vi "GetOutputShapeDimCount.vi"(8 "error in (no error)":errorcluster, 10 "outputIndex":i32, 11 "session id in":i32) -> (0 "error out":errorcluster, 2 "OutputShapeDimCount":i32, 3 "session id out":i32)   [LabVIEW 2017, in "libonnx_wrapper.lvlib"]
doc: "/**\n * @brief Получить количество размерностей выходного тензора\n * \n * Возвращает ранг тензора (число измерений). Например:\n * - Вектор [10] имеет 1 размерность\n * - Матрица [1, 10] имеет 2 размерности\n * - Изображение [1, 3, 224, 224] имеет 4 размерности\n * \n * @param sessionId [IN] ID сессии\n * @param outputIndex [IN] Индекс входа (0-based)\n * \n * @return int32: Количество размерностей (1, 2, 3, 4, ...)\n * @return int32: 0 если сессия не найдена или индекс неверен\n */\nint GetOutputShapeDimCount(int sessionId, int outputIndex);"
uses:
  libonnx_wrapper.lvlib
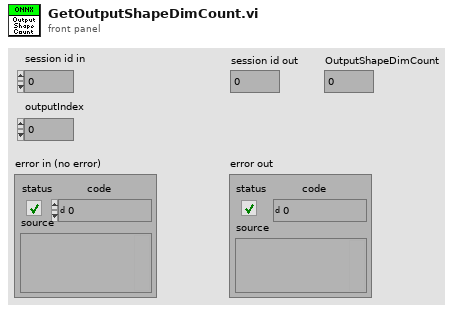
[diagram p1: front panel]
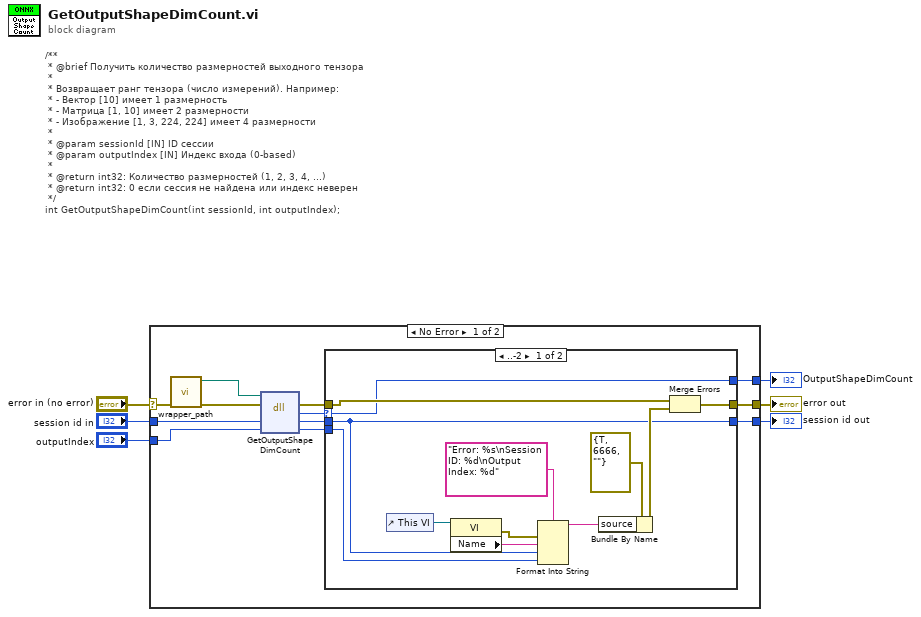
[diagram p0: block diagram]
diagram:
  # "/**\n * @brief Получить количество размерностей выходного тензора\n * \n * Возвращает ранг тензора (число измерений). Например:\n * - Вектор [10] имеет 1 размерность\n * - Матрица [1, 10] имеет 2 размерности\n * - Изображение [1, 3, 224, 224] имеет 4 размерности\n * \n * @param sessionId [IN] ID сессии\n * @param outputIndex [IN] Индекс входа (0-based)\n * \n * @return int32: Количество размерностей (1, 2, 3, 4, ...)\n * @return int32: 0 если сессия не найдена или индекс неверен\n */\nint GetOutputShapeDimCount(int sessionId, int outputIndex);"
  n1 = case shown="No Error" "error in (no error)" {
    selector: "error in (no error)" -> [w7 w35]
    tunnel: "outputIndex" -> [w18 _]
    tunnel: "session id in" -> [w16 w34]
    tunnel: [w13 w35] -> w4
    tunnel: [w11 _] -> w3
    tunnel: [w10 w34] -> w2
    frame No Error {
      n2 = call "wrapper_path.vi"("error in (no error)"=w7) -> ("error out"=w15:errorcluster, "wrapper path"=w17:path)  [unwired: 9 in]
      n3 = dll-call lib="home/ivan/LabVIEWData/ONNX/Test/libonnx_wrapper/unix64/libonnx_wrapper.so" fn="GetOutputShapeDimCount"(path in=w17, error in=w15, "sessionId"=w16, "inputIndex"=w18) -> (error out=w14:errorcluster, "return"=w12:i32, "sessionId"=w9:i32, "inputIndex"=w8:i32)  [unwired: 1 in, 1 out]
      n4 = case shown="..-2" w12 {
        selector: w12 -> [w19 w31]
        tunnel: w14 -> [w21 w33]
        tunnel: [w22 w33] -> w13
        tunnel: w9 -> [w23 w32]
        tunnel: [w23 w32] -> w10
        tunnel: w8 -> [w20 _]
        tunnel: [w19 w31] -> w11
        frame ..-2 {
          n5 = control-ref of="This VI"() -> (w27:refnum<vi>)
          n6 = property class="VI"(reference=w27) -> (error out=w24:errorcluster, "Name"=w26:string)  [unwired: 1 in, 1 out]
          n7 = Format Into String(format string="Error: %s\nSession ID: %d\nOutput Index: %d", error in=w24, w26, w23, w20) -> (resulting string=w28:string)  [unwired: 1 in, 1 out]
          n8 = Bundle By Name(cluster=errorcluster {"status"=TRUE, "code"=6666, "source"=""} ("error out"), "source"=w28) -> (w29:errorcluster)
          n9 = Merge Errors(w21, w29) -> (w22:errorcluster)
        }
        frame -1.. {
        }
      }
    }
    frame Error {
    }
  }
  "error out" <- w4
  "session id out" <- w2
  "OutputShapeDimCount" <- w3
